vi "Periodic Tasks.vi"(8 "error in":errorcluster) -> ()   [LabVIEW 2012]
doc: "This VI runs in parallel to other tasks. It can contain as many user-defined periodic loops as you need. These can carry out PID or other sorts of timed response."
uses:
  <vilib>/Rock Robotics/SystemInterfaces/Utilities/FPGA_UtilitiesLED Source.ctl
  <vilib>/Rock Robotics/SystemInterfaces/Utilities/FPGA_UtilitiesLED State.ctl
  Robot Global Data.vi
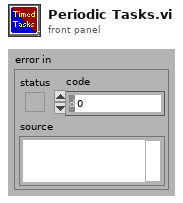
[diagram p1: front panel]
types:
  T1 = typedef "FPGA_UtilitiesLED State.ctl" = enum16{"Off", "On", "Toggle"}
  T2 = typedef "FPGA_UtilitiesLED Source.ctl" = enum16{"User LED", "FPGA LED"}
  T3 = typedef "WPI_JoystickDevRef.ctl" = cluster{"Device":T4}
  T4 = typedef "WPI_JoystickDeviceEnum.ctl" = enum16{"USB 1", "USB 2", "USB 3", "USB 4", "Kinect 1", "Kinect 2"}
  T5 = typedef "WPI_EncoderDevRef.ctl" = cluster{"DevStatus":errorcluster, "EncoderIndex":T6, "CounterIndex":T7, "DistancePerCount":dbl, "Decoding Type":T8}
  T6 = typedef "FPGA_EncoderIdx.ctl" = enum8{"Enc 0", "Enc 1", "Enc 2", "Enc 3", "Invalid"}
  T7 = typedef "FPGA_CounterCtrSystemIndex.ctl" = enum8{"Ctr 0", "Ctr 1", "Ctr 2", "Ctr 3", "Ctr 4", "Ctr 5", "Ctr 6", "Ctr 7", "Invalid"}
  T8 = typedef "WPI_EncoderType.ctl" = enum16{"1x", "2x", "4x"}
  T9 = typedef "WPI_JoystickButtonState.ctl" = cluster{"Button 1":bool, "Button 2":bool, "Button 3":bool, "Button 4":bool, "Button 5":bool, "Button 6":bool, "Button 7":bool, "Button 8":bool, "Button 9":bool, "Button 10":bool, "Button 11":bool, "Button 12":bool}
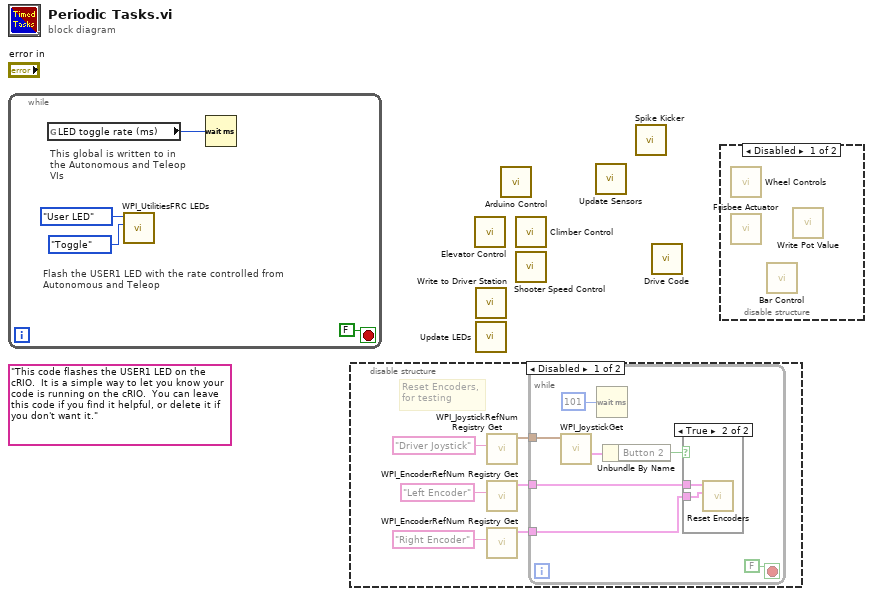
[diagram p0: block diagram]
diagram:
  (unwired) "This code flashes the USER1 LED on the cRIO.  It is a simple way to let you know your code is running on the cRIO.  You can leave this code if you find it helpful, or delete it if you don't want it."
  n1 = while {
    stop <- FALSE stop-if-true
    # "This global is written to in the Autonomous and Teleop VIs"
    # "Flash the USER1 LED with the rate controlled from Autonomous and Teleop"
    n2 = global read "Robot Global Data.vi" "LED toggle rate (ms)"() -> (w1:u32)
    n3 = call <vilib>:"WPI_UtilitiesFRC LEDs.vi"("State"=FPGA_UtilitiesLED_State."Toggle", "LED Type"=FPGA_UtilitiesLED_Source."User LED") -> ()  [unwired: 1 in, 9 out]
    n4 = Wait (ms)(milliseconds to wait=w1) -> ()  [unwired: 1 out]
  }
  n5 = disable-structure shown="Disabled" {
    frame Disabled {
      # "Reset Encoders,\nfor testing"
      n6 = call <vilib>:"WPI_JoystickRefNum Registry Get.vi"("refnum name"="Driver Joystick") -> ("JoystickDevRef"=w6:T3)  [unwired: 9 in, 1 out]
      n7 = call <vilib>:"WPI_EncoderRefNum Registry Get.vi"("refnum name"="Left Encoder") -> ("EncoderDevRef"=w9:T5)  [unwired: 9 in, 1 out]
      n8 = call <vilib>:"WPI_EncoderRefNum Registry Get.vi"("refnum name"="Right Encoder") -> ("EncoderDevRef"=w7:T5)  [unwired: 9 in, 1 out]
      n9 = while {
        tunnel: w9 -> [w15]
        tunnel: w7 -> [w14]
        tunnel: w6 -> [w13]
        stop <- FALSE stop-if-true
        n10 = call <vilib>:"WPI_JoystickGet.vi"("JoystickDevRef"=w13) -> ("Buttons"=w12:T9)  [unwired: 4 in, 2 out]
        n11 = Wait (ms)(milliseconds to wait=u32 101) -> ()  [unwired: 1 out]
        n12 = Unbundle By Name(w12) -> ("Button 2"=w11:bool)
        n13 = case shown="True" w11 {
          tunnel: w15 -> [_ w19]
          tunnel: w14 -> [_ w18]
          frame False {
          }
          frame True {
            n14 = call "Reset Encoders.vi"("Right Encoder"=w18, "Left Encoder"=w19) -> ()  [unwired: 10 in]
          }
        }
      }
    }
    frame Enabled {
    }
  }
  n15 = call "Elevator Control.vi"() -> ()  [unwired: 10 in, 2 out]
  n16 = call "Write to Driver Station.vi"() -> ()  [unwired: 12 in]
  n17 = call "Update LEDs.vi"() -> ()  [unwired: 12 in]
  n18 = call "Arduino Control.vi"() -> ()  [unwired: 12 in]
  n19 = call "Climber Control.vi"() -> ()  [unwired: 12 in]
  n20 = call "Shooter Speed Control.vi"() -> ()  [unwired: 8 in, 4 out]
  n21 = call "Update Sensors.vi"() -> ()  [unwired: 11 in, 1 out]
  n22 = call "Spike Kicker.vi"() -> ()  [unwired: 12 in]
  n23 = call "Drive Code.vi"() -> ()  [unwired: 12 in]
  n24 = disable-structure shown="Disabled" {
    frame Disabled {
      n25 = call "Wheel Controls.vi"() -> ()  [unwired: 12 in]
      n26 = call "Frisbee Actuator.vi"() -> ()  [unwired: 12 in]
      n27 = call "Bar Control.vi"() -> ()  [unwired: 12 in]
      n28 = call "Write Pot Value.vi"() -> ()  [unwired: 12 in]
    }
    frame Enabled {
    }
  }
